vi "Read DAQmx Config.vi"(8 "error in (no error)":errorcluster, 9 "data":T2, 11 "configuration file path":path) -> (0 "error out":errorcluster, 1 "DAQmx Chanel":T1, 3 "configuration file path out":path)   [LabVIEW 2020]
doc: "Odczytuje z pliku ustawienia akwizycji dla karty DAQ"
uses:
  <vilib>/Utility/config.llb/NI_LVConfig.lvlib
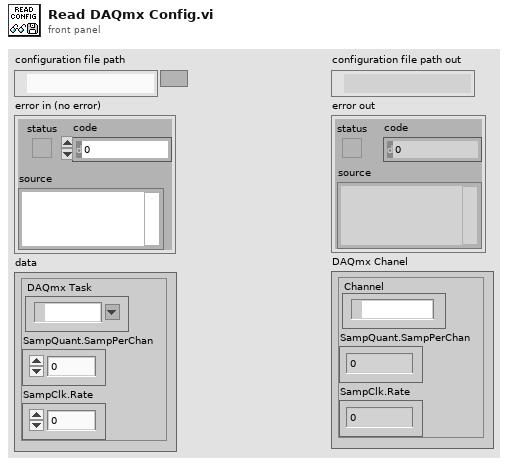
[diagram p1: front panel]
types:
  T1 = cluster{"SampClk.Rate":dbl, "SampQuant.SampPerChan":i32, "Channel":refnum<k21>}
  T2 = cluster{"SampClk.Rate":dbl, "SampQuant.SampPerChan":i32, "DAQmx Task":refnum<k21>}
  T3 = typedef "NI_LVConfig.lvlib/Config Data RefNum.ctl" = refnum<k1>
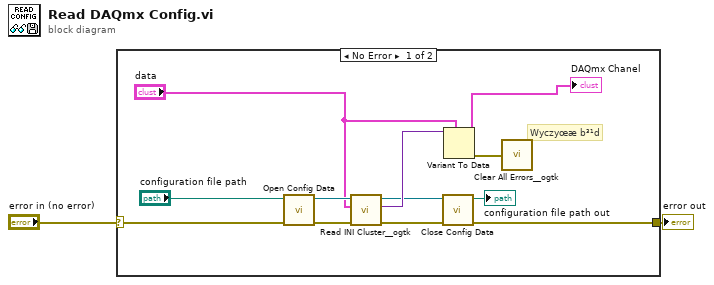
[diagram p0: block diagram]
diagram:
  n1 = case shown="No Error" "error in (no error)" {
    selector: "error in (no error)" -> [w7 w15]
    tunnel: [w8 w15] -> w2
    frame No Error {
      # "Wyczyœæ b³¹d"
      n2 = call <vilib>:"Open Config Data.vi"("error in (no error)"=w7, "configuration file path"="configuration file path") -> ("error out"=w14:errorcluster, "refnum"=w12:T3)  [unwired: 7 in, 1 out]
      n3 = call <userlib>:"Read INI Cluster__ogtk.vi"("error in (no error)"=w14, "INI Fomatted Cluster Type"="data", "refnum"=w12) -> ("error out"=w10:errorcluster, "INI Fomatted Cluster"=w11:variant, "dup refnum"=w9:T3)  [unwired: 4 in, 2 out]
      n4 = call <vilib>:"Close Config Data.vi"("error in (no error)"=w10, "refnum"=w9) -> ("error out"=w8:errorcluster, "file path"=→"configuration file path out":path)  [unwired: 8 in]
      n5 = Variant To Data(type="data", Variant=w11) -> (data=→"DAQmx Chanel":T2, error out=w5:errorcluster)  [unwired: 1 in]
      n6 = call <userlib>:"Clear All Errors__ogtk.vi"("Upsteam Error (optional)"=w5, "Error In"=w5) -> ()  [unwired: 2 in, 1 out]
    }
    frame Error {
    }
  }
  "error out" <- w2
